vi "ATF-Error FGV  RT Pump.vi"(7 "Enum":enum16{"Read", "Write", "Clear"}(ring), 11 "CS err":T1) -> (3 "CS err":T1)   [LabVIEW 2022 SP3]
panel:
  out "s? t:f":string
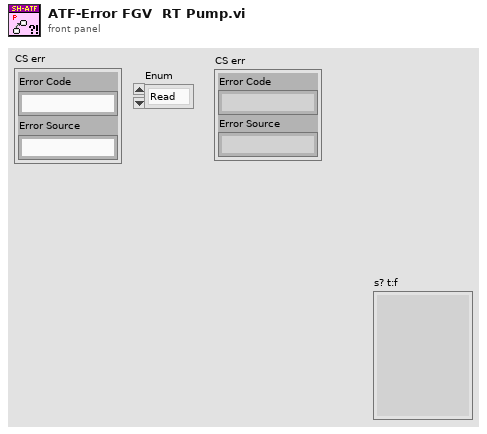
[diagram p1: front panel]
types:
  T1 = cluster{"Error Code":string, "Error Source":string}
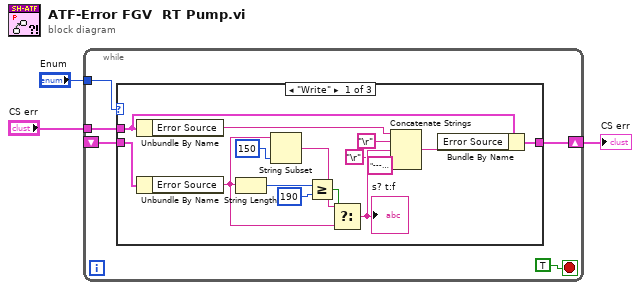
[diagram p0: block diagram]
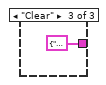
[diagram p3: hidden frame]
diagram:
  n1 = while {
    tunnel: "Enum" -> [w8]
    tunnel: "CS err" -> [w7]
    shift-right: [w6] -> w3
    shift-left: _ -> [w5]
    stop <- TRUE stop-if-true
    n2 = case shown="\"Write\"" w8 {
      tunnel: w7 -> [w20 _ _]
      tunnel: [w21 w24 T1 {"Error Code"="", "Error Source"=""} ("RT Error")] -> w6
      tunnel: w5 -> [w13 w24 _]
      frame "Write" {
        n3 = Unbundle By Name(w20) -> ("Error Source"=w23:string)
        n4 = Unbundle By Name(w13) -> ("Error Source"=w11:string)
        n5 = String Length(string=w11) -> (length=w17:i32)
        n6 = String Subset(string=w11, length (rest)=150 ("length (rest)")) -> (substring=w14:string)  [unwired: 1 in]
        n7 = Greater Or Equal?(x=w17, y=190) -> (x >= y?=w18:bool)
        n8 = Select(t=w14, s=w18, f=w11) -> (s? t:f=w12:string)
        "s? t:f" <- w12
        n9 = Concatenate Strings(w23, "\r", w12, "\r", "------------" ("string")) -> (w22:string)
        n10 = Bundle By Name(cluster=w20, "Error Source"=w22) -> (w21:T1)
      }
      frame "Read", Default {
      }
      frame "Clear" {
      }
    }
  }
  "CS err" <- w3
